vi "Set Plot Type.vi"(8 "error in (no error)":errorcluster, 10 "Plot type":T1, 11 "XY WFRM Plot in":refnum<class "XY WFRM Plot.lvclass">) -> (0 "error out":errorcluster, 3 "XY WFRM Plot out":refnum<class "XY WFRM Plot.lvclass">)   [LabVIEW 2018, in "XY WFRM Plot.lvclass"]
uses:
  XY WFRM Plot.lvclass
  Plot types.ctl
  XY WFRM Plot.lvclass/XY WFRM Plot.ctl
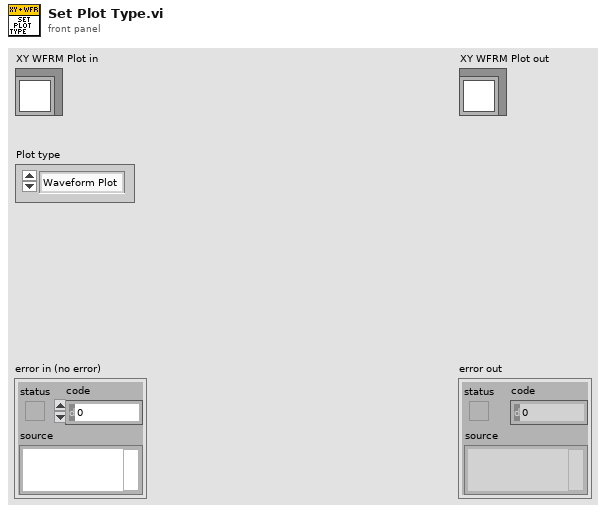
[diagram p1: front panel]
types:
  T1 = typedef "Plot types.ctl" = enum16{"Waveform Plot", "XY Plot", "Full XY"}
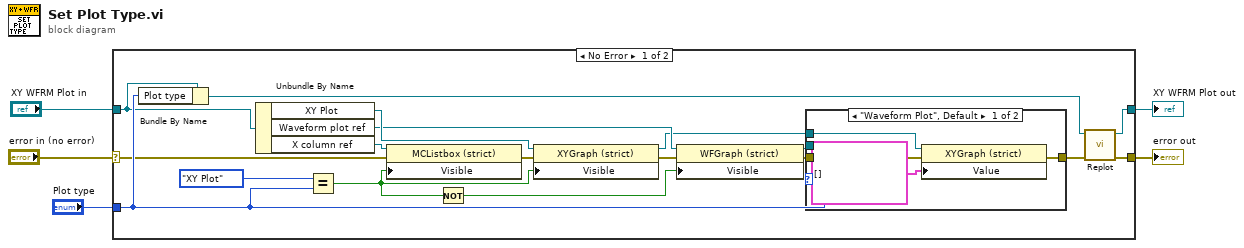
[diagram p0: block diagram]
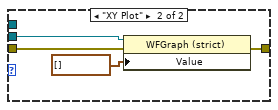
[diagram p2: hidden frame]
diagram:
  n1 = case shown="No Error" "error in (no error)" {
    selector: "error in (no error)" -> [w11 w33]
    tunnel: [w7 w33] -> w4
    tunnel: [w8 w32] -> w2
    tunnel: "XY WFRM Plot in" -> [w22 w32]
    tunnel: "Plot type" -> [w23 _]
    frame No Error {
      n2 = Bundle By Name(cluster=w22, "Plot type"=w23) -> (w21:refnum<class "XY WFRM Plot.lvclass">)
      n3 = Unbundle By Name(w22) -> ("XY Plot"=w20:refnum<vi>, "Waveform plot ref"=w19:refnum<vi>, "X column ref"=w10:refnum<vi>)
      n4 = Equal?(x=Plot_types."XY Plot" ("Plot type"), y=w23) -> (x = y?=w9:bool)
      n5 = property class="MCListbox (strict)"(reference=w10, error in=w11, "Visible"=w9) -> (error out=w12:errorcluster)  [unwired: 1 out]
      n6 = Not(x=w9) -> (.not. x?=w18:bool)
      n7 = property class="XYGraph (strict)"(reference=w20, error in=w12, "Visible"=w9) -> (reference out=w14:refnum<vi>, error out=w17:errorcluster)
      n8 = property class="WFGraph (strict)"(reference=w19, error in=w17, "Visible"=w18) -> (reference out=w15:refnum<vi>, error out=w16:errorcluster)
      n9 = case shown="\"Waveform Plot\", Default" w23 {
        tunnel: w16 -> [w27 w31]
        tunnel: w15 -> [_ w30]
        tunnel: [w26 w29] -> w6
        tunnel: w14 -> [w25 _]
        frame "Waveform Plot", Default {
          n10 = property class="XYGraph (strict)"(reference=w25, error in=w27, "Value"=cluster{"Y":dbl[], "Y":dbl[]}[] []) -> (error out=w26:errorcluster)  [unwired: 1 out]
        }
        frame "XY Plot" {
          n11 = property class="WFGraph (strict)"(reference=w30, error in=w31, "Value"=waveform(sgl)[] []) -> (error out=w29:errorcluster)  [unwired: 1 out]
        }
      }
      n12 = call-dynamic "Replot.vi"("error in (no error)"=w6, "Plot in"=w21) -> ("error out"=w7:errorcluster, "Plot out"=w8:refnum<class "XY WFRM Plot.lvclass">)  [unwired: 8 in]
    }
    frame Error {
    }
  }
  "error out" <- w4
  "XY WFRM Plot out" <- w2
